vi "ViewInsertVI.vi"(9 "UpdateInsertableVI":T1[](array[typedef]), 10 "Name":string, 11 "TabControl in":refnum<vi>) -> ()   [LabVIEW 2020]
uses:
  Ctl/UpdateInsertableVICtl.ctl
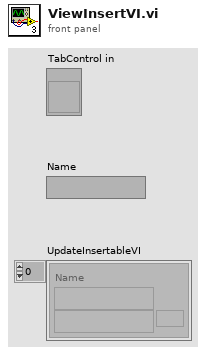
[diagram p1: front panel]
types:
  T1 = typedef "UpdateInsertableVICtl.ctl" = cluster{"Name":string, "VIPath":path}
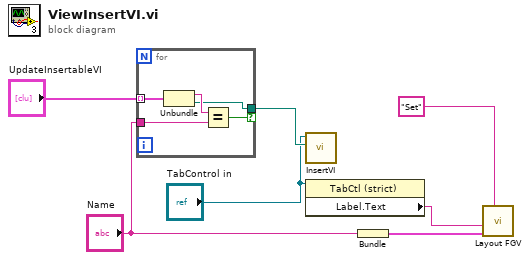
[diagram p0: block diagram]
diagram:
  n1 = for {
    tunnel: "UpdateInsertableVI" -> [w11] mode=indexing
    tunnel: "Name" -> [w12]
    tunnel: [w9] -> w6 if=w8
    n2 = Unbundle(w11) -> ("Name"=w10:string, "VIPath"=w9:path)
    n3 = Equal?(x=w10, y=w12) -> (x = y?=w8:bool)
  }
  n4 = call "InsertVI.vi"("VIPath"=w6, "TabControl in"="TabControl in") -> ()  [unwired: 9 in, 1 out]
  n5 = property class="TabCtl (strict)"(reference="TabControl in") -> ("Label.Text"=w4:string)  [unwired: 1 in, 2 out]
  n6 = Bundle("Name"="Name") -> (w3:cluster{"Name":string})  [unwired: 1 in]
  n7 = call "Layout FGV.vi"("String"="Set", "Variant"=w3, "name"=w4) -> ()  [unwired: 9 in]
